vi "Intan_SaveDisplayData.vi"(3 "2d ADCdata_array out":dbl[][](array[numeric]), 4 "byte order  2":T1(ring)=enum."little-endian", 5 "aux file ref num":refnum<file>) -> (2 "refnum out":refnum<file>)   [LabVIEW 2017]
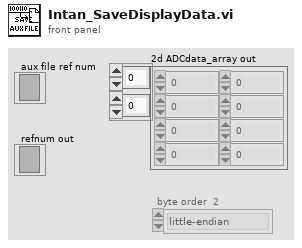
[diagram p1: front panel]
types:
  T1 = enum16{"big-endian, network order", "native, host order", "little-endian"}
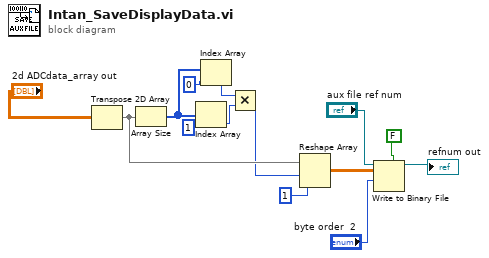
[diagram p0: block diagram]
diagram:
  n1 = Transpose 2D Array(2D array="2d ADCdata_array out") -> (transposed array=w5:dbl[][])
  n2 = Array Size(array=w5) -> (size(s)=w11:i32[])
  n3 = Index Array(array=w11, index=1) -> (element=w7:i32)
  n4 = Index Array(array=w11, index=0) -> (element=w8:i32)
  n5 = Multiply(x=w8, y=w7) -> (x*y=w3:i32)
  n6 = Reshape Array(w5, w3, 1 ("dimension size")) -> (w6:dbl[][])
  n7 = Write to Binary File(file (use dialog)="aux file ref num", data=w6, 5:FALSE ("prepend array or string size? (T)"), 9:"byte order  2") -> (refnum out=→"refnum out":refnum<file>)  [unwired: 2 in, 2 out]
